vi "Helper_JSON (SubVI).vi"(8 "error in (no error)":errorcluster, 9 "Inner JSON":string="result", 10 "Outer JSON":string="rows", 11 "body":string) -> (0 "error out":errorcluster, 3 "String Value":string)   [LabVIEW 2018]
uses:
  <vilib>/LVH/i3 JSON/JSON Parsing/Get Object Parameter Files/Get Object Parameter - Array.vi
  <vilib>/LVH/i3 JSON/JSON Parsing/Get Array Value at Index Files/Get Array Value at Index - Object.vi
  <vilib>/LVH/i3 JSON/JSON Parsing/Get Object Parameter Files/Get Object Parameter - String.vi
  <vilib>/LVH/i3 JSON/i3-json.lvlib
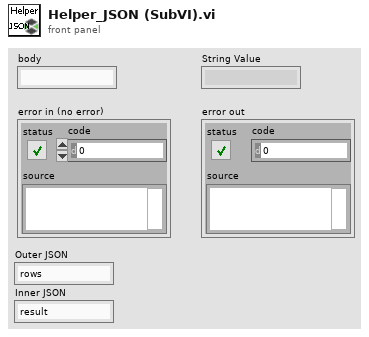
[diagram p1: front panel]
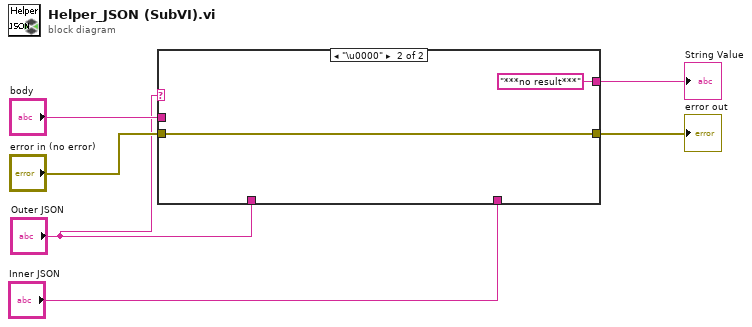
[diagram p0: block diagram]
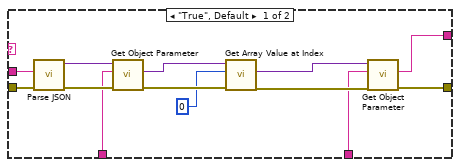
[diagram p2: hidden frame]
diagram:
  n1 = case shown="\"\"" "Outer JSON" {
    tunnel: [w19 w21] -> w6
    tunnel: [w15 "***no result***" ("String Value")] -> w5
    tunnel: "Inner JSON" -> [w13 _]
    tunnel: "Outer JSON" -> [w10 _]
    tunnel: "body" -> [w8 _]
    tunnel: "error in (no error)" -> [w7 w21]
    frame "True", Default {
      n2 = call <vilib>:"Parse JSON.vi"("error in (no error)"=w7, "JSON String"=w8) -> ("error out"=w16:errorcluster, "JSON Tree"=w9:variant)  [unwired: 6 in, 2 out]
      n3 = call-poly <vilib>:"Get Object Parameter.vi"("error in (no error)"=w16, "Parameter Name"=w10, "JSON Tree In (JSON Object)"=w9) -> ("error out"=w17:errorcluster, "JSON Array"=w11:variant)  [unwired: 5 in, 2 out]
      n4 = call-poly <vilib>:"Get Array Value at Index.vi"("error in (no error)"=w17, "Index"=0, "JSON Tree In (JSON Array)"=w11) -> ("error out"=w18:errorcluster, "JSON Object"=w14:variant)  [unwired: 5 in, 2 out]
      n5 = call-poly <vilib>:"Get Object Parameter.vi"("error in (no error)"=w18, "Parameter Name"=w13, "JSON Tree In (JSON Object)"=w14) -> ("error out"=w19:errorcluster, "String Value"=w15:string)  [unwired: 5 in, 2 out]
    }
    frame "\u0000" {
    }
  }
  "error out" <- w6
  "String Value" <- w5
